vi "Get Source Value.vi"(8 "error in (no error)":errorcluster, 11 "Stanford Research PS350 in":refnum<class "Stanford Research PS350.lvclass">) -> (0 "error out":errorcluster, 2 "Source Value":dbl, 3 "Stanford Research PS350 out":refnum<class "Stanford Research PS350.lvclass">, 5 "Source Value Units":T1)   [LabVIEW 2011, in "Stanford Research PS350.lvclass"]
uses:
  Stanford Research PS350.lvclass
  Power Supply/Source Units.ctl
  Stanford Research PS350.lvclass/Stanford Research PS350.ctl
  Power Supply/Power Supply.lvclass
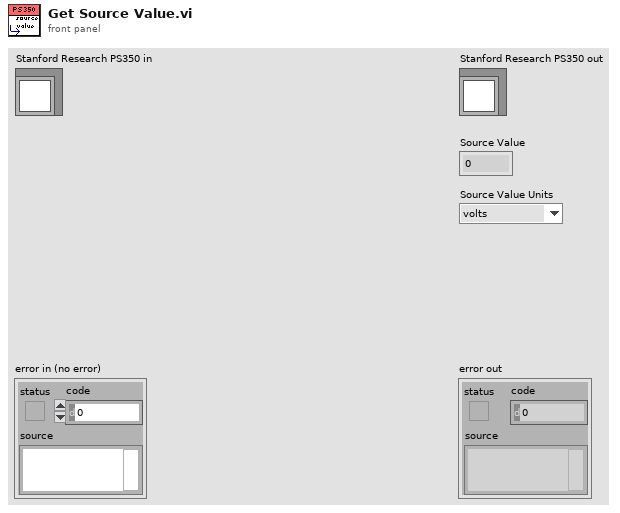
[diagram p1: front panel]
types:
  T1 = typedef "Power Supply.lvclass/Source Units.ctl" = enum16{"volts", "millivolts", "microvolts", "amps", "milliamps", "microamps", "nanoamps"}
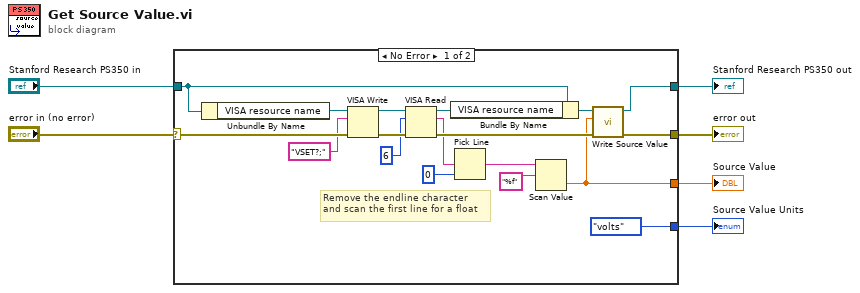
[diagram p0: block diagram]
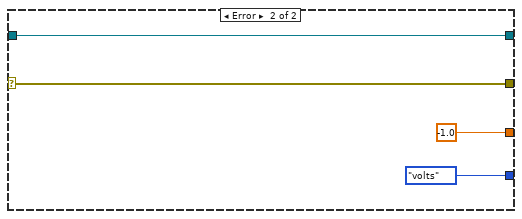
[diagram p2: hidden frame]
diagram:
  n1 = case shown="No Error" "error in (no error)" {
    selector: "error in (no error)" -> [w17 w28]
    tunnel: [w22 w28] -> w5
    tunnel: [w21 w27] -> w3
    tunnel: "Stanford Research PS350 in" -> [w24 w27]
    tunnel: [Source_Units."volts" ("Source Value Units") Source_Units."volts" ("Source Value Units")] -> w2
    tunnel: [w8 -1.0] -> w1
    frame No Error {
      # "Remove the endline character\nand scan the first line for a float"
      n2 = Unbundle By Name(w24) -> ("VISA resource name"=w20:refnum<visa-resource-name>)
      n3 = VISA Write(VISA resource name=w20, write buffer="VSET?;", error in (no error)=w17) -> (VISA resource name out=w19:refnum<visa-resource-name>, error out=w16:errorcluster)  [unwired: 1 out]
      n4 = VISA Read(VISA resource name=w19, byte count=u32 6, error in (no error)=w16) -> (VISA resource name out=w18:refnum<visa-resource-name>, read buffer=w11:string, error out=w15:errorcluster)  [unwired: 1 out]
      n5 = Bundle By Name(cluster=w24, "VISA resource name"=w18) -> (w23:refnum<class "Stanford Research PS350.lvclass">)
      n6 = Pick Line(multi-line string=w11, line index=0) -> (output string=w10:string)  [unwired: 1 in]
      n7 = Scan Value(string=w10, format string="%f") -> (value=w8:dbl)  [unwired: 1 in, 1 out]
      n8 = call-dynamic "Write Source Value.vi"("error in (no error)"=w15, "Source Value"=w8, "Power Supply in"=w23) -> ("error out"=w22:errorcluster, "Power Supply out"=w21:refnum<class "Stanford Research PS350.lvclass">)  [unwired: 7 in]
    }
    frame Error {
    }
  }
  "error out" <- w5
  "Stanford Research PS350 out" <- w3
  "Source Value Units" <- w2
  "Source Value" <- w1
